vi "Guardians Check Infinite Message.vi"(6 "Infinite Message Selector":T1, 8 "error in (no error)":errorcluster, 11 "Guardian in":refnum<class "Guardian.lvclass">) -> (0 "error out":errorcluster, 2 "Exists?":bool, 3 "Guardian out":refnum<class "Guardian.lvclass">)   [LabVIEW 2026, in "TALOS.lvlib" / "Guardian.lvlib" / "Guardian.lvclass"]
doc: "This VI start the infinite messaging to periodically check the status of the Guardians. It grabs the notifier so to be able to stop it afterwards."
uses:
  Guardian.lvclass
  Ancestor/Ancestor/Infinite Message Selector.ctl
  Guardian Messages/Guardians Status Check Msg/Guardians Status Check Msg.lvclass
  C:/LabVIEW Code/TALOS/builds/Actor Framework PPL/Actor Framework.lvlibp/1abvi3w/vi.lib/ActorFramework/Message/Message.lvclass
  Ancestor/Ancestor/Ancestor.lvclass/Ancestor.ctl
  Support VIs/Generate Error.vi
  FGV/Error Memory/Get Error Description.vi
  Support VIs/Get PC name.vi
  Ancestor/Ancestor/Read ID.vi
  Support VIs/Get Class Name.vi
  FGV/Error Memory/Error Memory Core.vi
  <vilib>/AdvancedString/Delimited String to 1D String Array.vi
  <vilib>/AdvancedString/Delimited String to 1D String Array (string).vi
  Support VIs/Circus Root Path.vi
  FGV/Error Memory/Error Crt Lvl checker.vi
  FGV/Error Memory/Error Memory Core.vi/40c8088d-b597-4017-91af-faa98e00292e.vi
  FGV/Error Memory/Error Memory Core.vi/d4a3ab98-063c-4e44-b43d-fbdcfe6c2be2.vi
  Support VIs/Global Memory.vi
  <vilib>/Utility/LVClass/Get LV Class Name.vi
  Support VIs/Is in Packed Library.vi
  Support VIs/TALOS Root path.vi
  Support VIs/Read CSV worksheet.vi
  Support VIs/Global Constants.vi
  <vilib>/Utility/error.llb/General Error Handler.vi
  Support VIs/Error Log.vi
  Ancestor/Ancestor/Ancestor.lvclass
  <vilib>/Comparison/Equal/Equal Functor/Equal Functor.lvclass
  TALOS.lvlib
  <userlib>/_OpenG.lib/lvdata/lvdata.llb/openg_variant.lvlib
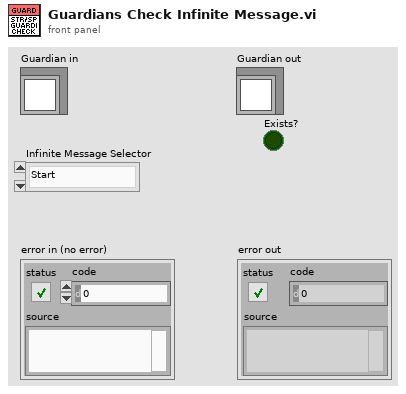
[diagram p1: front panel]
types:
  T1 = typedef "TALOS.lvlib/Ancestor.lvlib/Ancestor.lvclass/Infinite Message Selector.ctl" = enum16{"Start", "Stop", "Check", "Flush (Stop all)", "Init"}
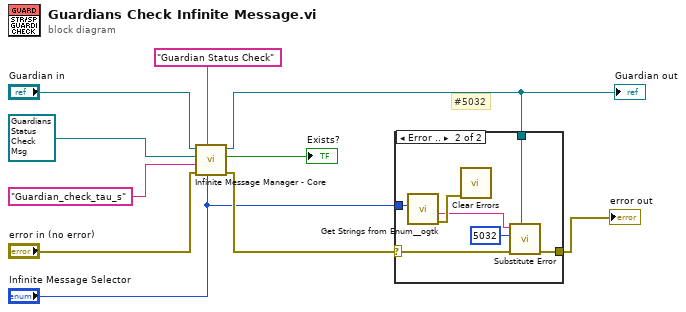
[diagram p0: block diagram]
diagram:
  # "#5032"
  n1 = call-dynamic "Infinite Message Manager - Core.vi"("Infinite Message Selector"="Infinite Message Selector", "Msg ID"="Guardian Status Check", "error in (no error)"="error in (no error)", "Tau parameter"="Guardian_check_tau_s" ("Parameter Name"), "Actor Framework:Message"=refnum<class "Guardians Status Check Msg.lvclass"> refnum ("TALOS.lvlib:Guardian.lvlib:Guardians Status Check Msg.lvclass"), "Ancestor in"="Guardian in") -> ("error out"=w4:errorcluster, "Exists?"=→"Exists?":bool, "Ancestor out"=w2:refnum<class "Guardian.lvclass">)  [unwired: 3 in]
  "Guardian out" <- w2
  n2 = case shown="Error .." w4 {
    selector: w4 -> [w11 w18]
    tunnel: [w11 w17] -> w1
    tunnel: w2 -> [_ w16]
    tunnel: "Infinite Message Selector" -> [_ w14]
    frame No Error {
    }
    frame Error {
      n3 = call <userlib>:"Get Strings from Enum__ogtk.vi"("Enum"=w14) -> ("error out"=w13:errorcluster, "String Value"=w12:string)  [unwired: 7 in, 2 out]
      n4 = call <vilib>:"Clear Errors.vi"("error in (no error)"=w13) -> ()  [unwired: 5 in, 2 out]
      n5 = call "Substitute Error.vi"("LabVIEW Object"=w16, "error in (no error)"=w18, "Error Code"=5032, "Optional String"=w12) -> ("error out"=w17:errorcluster)  [unwired: 7 in]
    }
  }
  "error out" <- w1
